vi "Atitude Control Test.vi"() -> ()   [LabVIEW 2012]
uses:
  <vilib>/Utility/miscctls.llb/LV3DPointTypeDef.ctl
  lv-attitudecontrol.lvlib
panel:
  in  "Attitude Indicator":refnum<vi>(3d-picture)
  in  "stop":bool
  in  "Control 1":T1 {"X" scale=-90.0..90.0; "Y" scale=-180.0..180.0; "Z" scale=0.0..360.0}
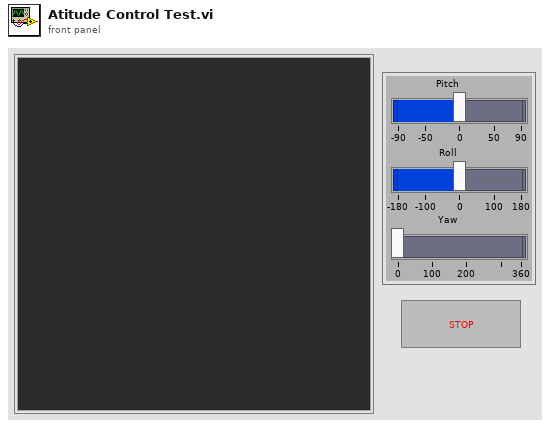
[diagram p1: front panel]
types:
  T1 = typedef "LV3DPointTypeDef.ctl" = cluster{"X":sgl, "Y":sgl, "Z":sgl}
  T2 = typedef "lv-attitudecontrol.lvlib/AttitudeHandle.ctl" = cluster{"First Scene Object":refnum<vi>, "Drum":refnum<vi>, "Window":refnum<vi>, "Dial":refnum<vi>, "Scene Graph":refnum<vi>, "Last Drum Pitch":dbl, "Last Drum Roll ":dbl, "Last Dial Roll":dbl}
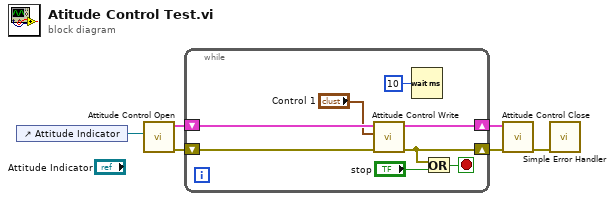
[diagram p0: block diagram]
diagram:
  n1 = control-ref of="Attitude Indicator"() -> (w4:refnum<vi>)
  n2 = call "Attitude Control Open.vi"("Scene Graph"=w4) -> ("error out"=w5:errorcluster, "Attitude Control Handle"=w6:T2)  [unwired: 9 in]
  n3 = while {
    shift-right: [w7] -> w2
    shift-left: w6 -> [w14]
    shift-right: [w8] -> w3
    shift-left: w5 -> [w13]
    stop <- w9 stop-if-true
    n4 = call "Attitude Control Write.vi"("error in (no error)"=w13, "pitch (x), roll (y), yaw (z)"="Control 1", "Attitude Control Handle In"=w14) -> ("error out"=w8:errorcluster, "Attitude Control Handle Out"=w7:T2)  [unwired: 7 in]
    n5 = Wait (ms)(milliseconds to wait=u32 10) -> ()  [unwired: 1 out]
    n6 = Or(x=w8, y="stop") -> (x .or. y?=w9:bool)
  }
  n7 = call "Attitude Control Close.vi"("error in (no error)"=w3, "Attitude Control Handle"=w2) -> ("error out"=w1:errorcluster)  [unwired: 9 in]
  n8 = call <vilib>:"Simple Error Handler.vi"("error in (no error)"=w1) -> ()  [unwired: 4 in, 5 out]
